vi "Car Wash.vi"() -> ()   [LabVIEW 8.6]
doc: "This VI allows you to simulate a car wash. The wash options controls allow you to determine which cycles will be performed. If none are selected, the High Pressure Wash cycle is the default. Once the start button is clicked, the wash begins. Use the Car Position Simulation control to simulate the position of the vehicle. If the vehicle is in the wrong position for the current cycle, the wash indicators will indicate that and you should change the car position. The Car wash display will give the current status of the wash cycle. The \"Stop Program\" button will stop the car wash immediately."
uses:
  Controls/State Control Enum.ctl
  Controls/Car Wash Indicators.ctl
  Controls/Car Position Control.ctl
  Controls/Wash Options.ctl
panel:
  in  "Stop":bool
  out "Elapsed Time (sec)":dbl format="%#.2g"
  out "Wash Indicators":T1
  in  "Car Position Slider":T2
  out "Wash Entry":bool
  in  "Start":bool
  in  "Wash Options":T3
  # "Entry Console"
  # "Car Wash Display"
  # "The wash options controls allow you to determine which cycles will be performed.  \n\nIf none are selected, the High Pressure Wash cycle is the default.  \n\nOnce the start button is clicked, the wash begins."
  # "The Wash Entry LED indicates whether or not the wash in vacant or in use.\n\nThe Wash Indicator LEDs indicate the current status when the wash is in use.\n\nThe Elapsed Time indicator shows the progress for the current cycle, only if it is a timed cycle."
  # "Car Position Simulation"
  # "The Car Position Slider allows you to simulate the position of a vehicle in the wash.\nThe vehicle must be at the correct station for the each wash cycle to work.  The cycles that are completed at each station are indicated below the station number.\nIf the Vehicle Out of Position LED above is green, adjust your position to the appropraite station."
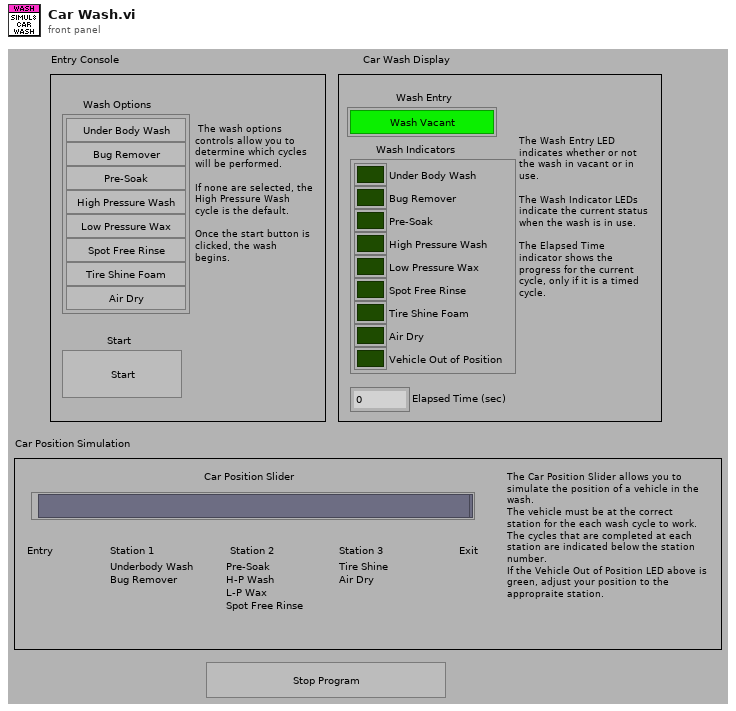
[diagram p1: front panel]
types:
  T1 = typedef "Car Wash Indicators.ctl" = cluster{"Under Body Wash":bool, "Bug Remover":bool, "Pre-Soak":bool, "High Pressure Wash":bool, "Low Pressure Wax":bool, "Spot Free Rinse":bool, "Tire Shine Foam":bool, "Air Dry":bool, "Vehicle Out of Position":bool}
  T2 = typedef "Car Position Control.ctl" = i32
  T3 = typedef "Wash Options.ctl" = cluster{"Under Body Wash":bool, "Bug Remover":bool, "Pre-Soak":bool, "High Pressure Wash":bool, "Low Pressure Wax":bool, "Spot Free Rinse":bool, "Tire Shine Foam":bool, "Air Dry":bool}
  T4 = typedef "State Control Enum.ctl" = enum16{"Initialize", "Wait for Start", "Underbody Wash", "Bug Remover", "Presoak", "HP Wash", "LP Wax", "Spot Free Rinse", "Tire Shine", "Air Dry", "Exit", "Skip", "Stop"}
  T5 = enum8{"Enabled", "Disabled", "Disabled and Grayed Out"}
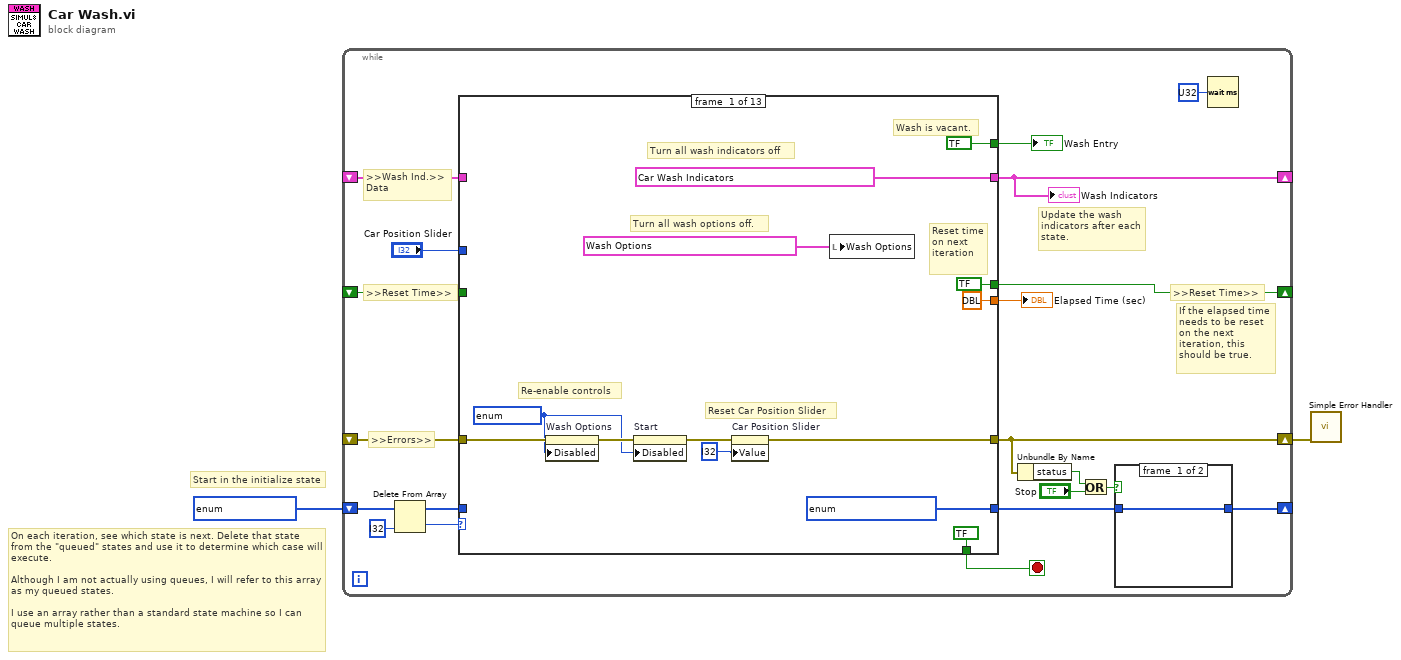
[diagram p0: block diagram]
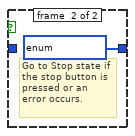
[diagram p2: hidden frame]
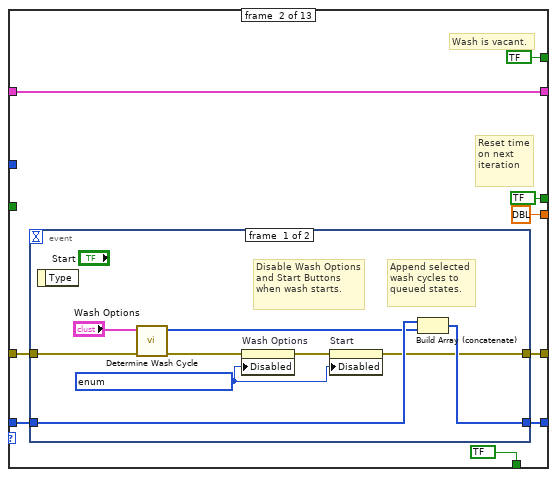
[diagram p3: hidden frame]
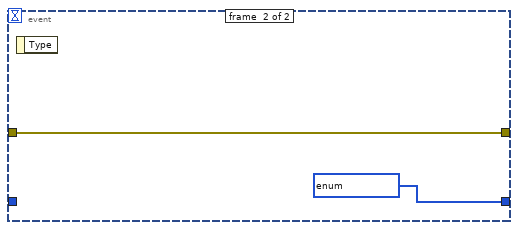
[diagram p4: hidden frame]
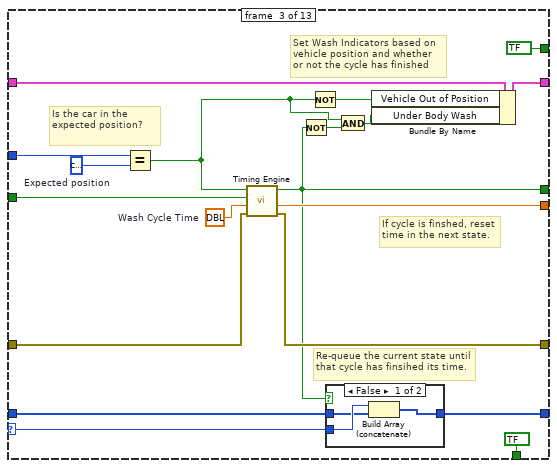
[diagram p5: hidden frame]
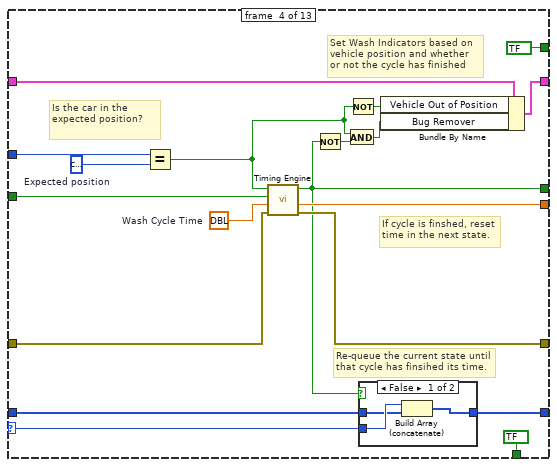
[diagram p7: hidden frame]
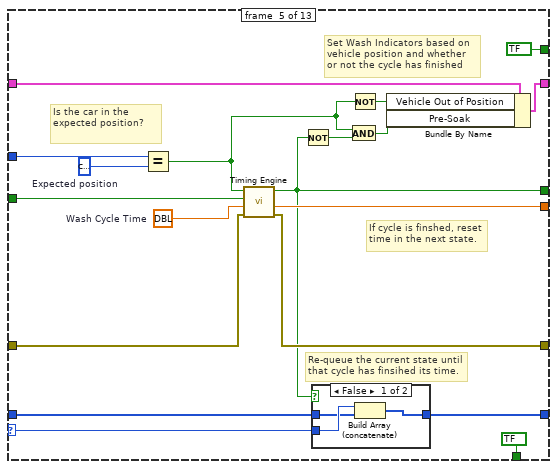
[diagram p9: hidden frame]
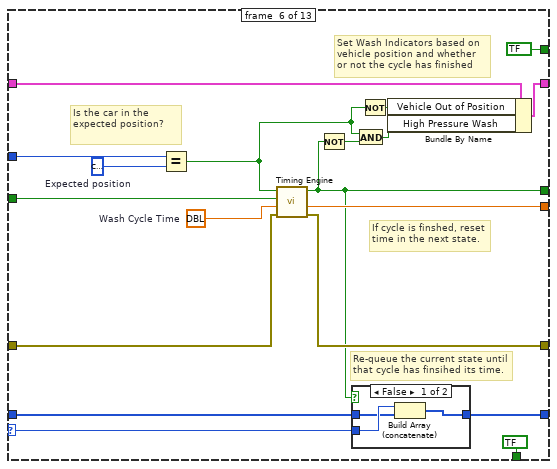
[diagram p11: hidden frame]
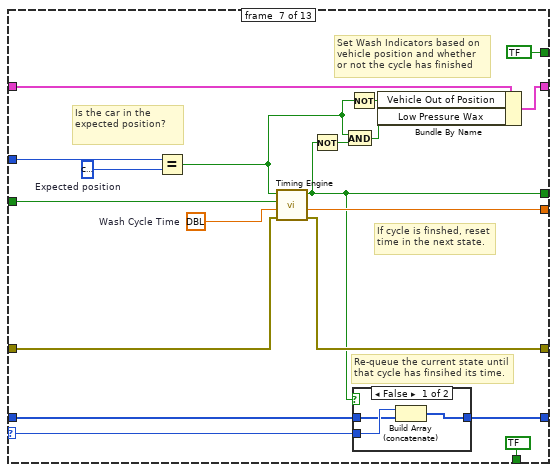
[diagram p13: hidden frame]
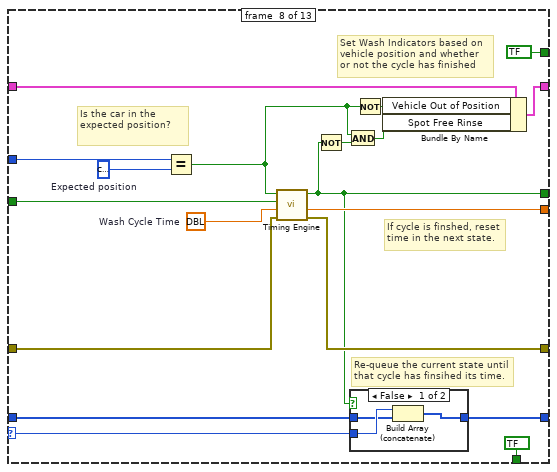
[diagram p15: hidden frame]
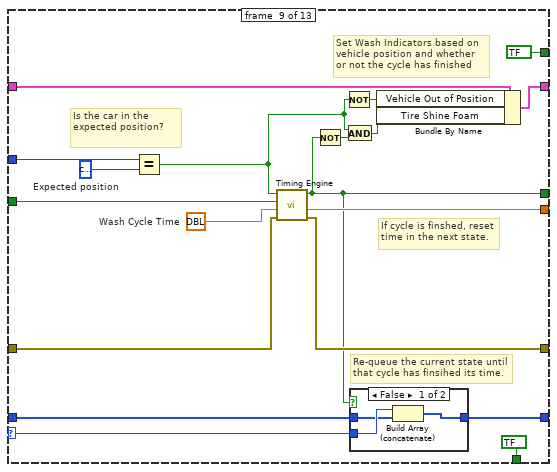
[diagram p17: hidden frame]
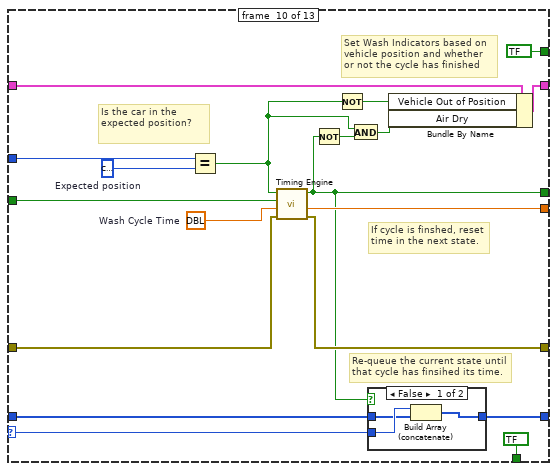
[diagram p19: hidden frame]
diagram:
  w2 = T4[] ? items=["Initialize", "Wait for Start", "Underbody Wash", "Bug Remover", "Presoak", "HP Wash", "LP Wax", "Spot Free Rinse", "Tire Shine", "Air Dry", "Exit", "Skip", "Stop"]
  # "Start in the initialize state"
  # "On each iteration, see which state is next. Delete that state from the \"queued\" states and use it to determine which case will execute. \n\nAlthough I am not actually using queues, I will refer to this array as my queued states.  \n\nI use an array rather than a standard state machine so I can queue multiple states."
  n1 = while {
    shift-right: [w14] -> _
    shift-left: w2 -> [w22]
    shift-right: [w17] -> _
    shift-left: _ -> [w18]
    shift-right: [w6] -> w1
    shift-left: _ -> [w13]
    shift-right: [w12] -> _
    shift-left: _ -> [w11]
    stop <- w8 stop-if-true
    # "Update the wash indicators after each state."
    # "If the elapsed time needs to be reset on the next iteration, this should be true."
    # ">>Reset Time>>"
    # ">>Errors>>"
    # ">>Wash Ind.>>\nData"
    # ">>Reset Time>>"
    n2 = Delete From Array(array=w22, index=i32 ?) -> (deleted portion=w19:T4, array with subset deleted=w20:T4[])  [unwired: 1 in]
    n3 = case shown="\"Air Dry\"" w19 {
      selector: w19 -> [_ _ w65 w90 w114 w143 w159 w188 w204 w232 _ _ _]
      tunnel: w20 -> [_ w44 w64 w91 w115 w142 w158 w187 w203 w231 _ w256 _]
      tunnel: [w29 w45 w66 w89 w113 w141 w157 w180 w205 w230 w243 w256 w270] -> w15
      tunnel: [T1 ? ("Wash Indicators 2") w38 w67 w92 w116 w135 w160 w184 w206 w233 T1 ? ("Wash Indicators 2") w253 w272] -> w17
      tunnel: w18 -> [_ w38 w68 w93 w117 w136 w161 w185 w207 w234 _ w253 w273]
      tunnel: [bool ? ("Wash Entry") bool ? ("Wash Entry") bool ? ("Wash Entry") bool ? ("Wash Entry") bool ? ("Wash Entry") bool ? ("Wash Entry") bool ? ("Wash Entry") bool ? ("Wash Entry") bool ? ("Wash Entry") bool ? ("Wash Entry") bool ? ("Wash Entry") bool ? ("Wash Entry") bool ? ("Wash Entry")] -> w16
      tunnel: w13 -> [w35 w43 w72 w95 w109 w139 w165 w181 w212 w228 w250 w257 w266]
      tunnel: [w25 w42 w73 w94 w110 w140 w164 w189 w211 w229 w249 w258 w266] -> w6
      tunnel: [bool ? ("Time Expired?") bool ? ("Wash Entry") w58 w84 w105 w128 w153 w176 w200 w221 bool ? ("Time Expired?") w260 bool ? ("Time Expired?")] -> w12
      tunnel: w11 -> [_ _ w75 w96 w119 w138 w162 w182 w210 w227 _ w260 _]
      tunnel: [dbl ? ("Elapsed Time") dbl ? ("Elapsed Time") w74 w86 w118 w134 w166 w186 w208 w235 dbl ? ("Elapsed Time") w262 dbl ? ("Elapsed Time")] -> w10
      tunnel: "Car Position Slider" -> [_ _ w70 w97 w120 w137 w163 w183 w209 w226 _ _ w264]
      tunnel: [bool ? ("Wash Entry") bool ? ("Wash Entry") bool ? ("Wash Entry") bool ? ("Wash Entry") bool ? ("Wash Entry") bool ? ("Wash Entry") bool ? ("Wash Entry") bool ? ("Wash Entry") bool ? ("Wash Entry") bool ? ("Wash Entry") bool ? ("Wash Entry") bool ? ("Wash Entry") bool ? ("Wash Entry")] -> w8
      frame #0 {
        w29 = T4[] ? items=["Initialize", "Wait for Start", "Underbody Wash", "Bug Remover", "Presoak", "HP Wash", "LP Wax", "Spot Free Rinse", "Tire Shine", "Air Dry", "Exit", "Skip", "Stop"]
        w26 = T5 ? ("Disabled")
        # "Reset time on next iteration"
        # "Re-enable controls"
        # "Reset Car Position Slider"
        # "Wash is vacant."
        # "Turn all wash indicators off"
        # "Turn all wash options off."
        n4 = property on="Wash Options" class="Clust (strict)"(error in=w35, "Disabled"=w26) -> (error out=w34:errorcluster)  [unwired: 1 in, 1 out]
        n5 = property on="Start" class="Bool"(error in=w34, "Disabled"=w26) -> (error out=w28:errorcluster)  [unwired: 1 in, 1 out]
        n6 = property on="Car Position Slider" class="Slide (strict)"(error in=w28, "Value"=i32 ?) -> (error out=w25:errorcluster)  [unwired: 1 in, 1 out]
        n7 = local write "Wash Options"(T3 ? ("Wash Options")) -> ()
      }
      frame #1 {
        # "Wash is vacant."
        # "Reset time on next iteration"
        n8 = event shown="[1] \"Stop\": Value Change" {
          selector: _ -> [_ _]
          dyn-events: _ -> [_ _]
          timeout: _ -> [_ _]
          tunnel: [w51 w57] -> w45
          tunnel: w44 -> [w53 _]
          tunnel: [w47 w56] -> w42
          tunnel: w43 -> [w48 w56]
          event #0 {
            w49 = T5 ? ("Disabled")
            # "Append selected wash cycles to queued states."
            # "Disable Wash Options and Start Buttons when wash starts."
            n9 = event-data() -> ()  [unwired: 1 in, 1 out]
            n10 = call "Determine Wash Cycle.vi"("error in"=w48, "Wash Options"="Wash Options") -> ("error out"=w54:errorcluster, "Wash Cycles"=w52:T4[])  [unwired: 8 in]
            n11 = property on="Wash Options" class="Clust (strict)"(error in=w54, "Disabled"=w49) -> (error out=w50:errorcluster)  [unwired: 1 in, 1 out]
            n12 = property on="Start" class="Bool"(error in=w50, "Disabled"=w49) -> (error out=w47:errorcluster)  [unwired: 1 in, 1 out]
            n13 = Build Array (concatenate)(w53, w52) -> (w51:T4[])
          }
          event #1 {
            w57 = T4[] ? items=["Initialize", "Wait for Start", "Underbody Wash", "Bug Remover", "Presoak", "HP Wash", "LP Wax", "Spot Free Rinse", "Tire Shine", "Air Dry", "Exit", "Skip", "Stop"]
            n14 = event-data() -> ()  [unwired: 1 in, 1 out]
          }
        }
      }
      frame #2 {
        w69 = T2 ?  # Expected position
        w71 = dbl ?  # Wash Cycle Time
        # "Is the car in the expected position?"
        # "Re-queue the current state until that cycle has finsihed its time."
        # "If cycle is finshed, reset time in the next state."
        # "Set Wash Indicators based on vehicle position and whether or not the cycle has finished"
        n15 = Equal?(x=w70, y=w69) -> (x = y?=w60:bool)
        n16 = call "Timing Engine.vi"("error in"=w72, "Time Limit"=w71, "Reset"=w75, "Advance Time?"=w60) -> ("error out"=w73:errorcluster, "Elapsed Time"=w74:dbl, "Time Expired?"=w58:bool)  [unwired: 5 in]
        n17 = Not(x=w58) -> (.not. x?=w61:bool)
        n18 = Not(x=w60) -> (.not. x?=w63:bool)
        n19 = case shown="False" w58 {
          tunnel: [w79 w80] -> w66
          tunnel: w65 -> [w78 _]
          tunnel: w64 -> [w77 w80]
          frame #0 {
            n20 = Build Array (concatenate)(w78, w77) -> (w79:T4[])
          }
          frame #1 {
          }
        }
        n21 = And(x=w60, y=w61) -> (x .and. y?=w59:bool)
        n22 = Bundle By Name(cluster=w68, "Vehicle Out of Position"=w63, "Under Body Wash"=w59) -> (w67:T1)
      }
      frame #3 {
        w81 = T2 ?  # Expected position
        w98 = dbl ?  # Wash Cycle Time
        # "Is the car in the expected position?"
        # "Re-queue the current state until that cycle has finsihed its time."
        # "If cycle is finshed, reset time in the next state."
        # "Set Wash Indicators based on vehicle position and whether or not the cycle has finished"
        n23 = Equal?(x=w97, y=w81) -> (x = y?=w83:bool)
        n24 = call "Timing Engine.vi"("error in"=w95, "Time Limit"=w98, "Reset"=w96, "Advance Time?"=w83) -> ("error out"=w94:errorcluster, "Elapsed Time"=w86:dbl, "Time Expired?"=w84:bool)  [unwired: 5 in]
        n25 = Not(x=w84) -> (.not. x?=w85:bool)
        n26 = And(x=w83, y=w85) -> (x .and. y?=w82:bool)
        n27 = Not(x=w83) -> (.not. x?=w88:bool)
        n28 = case shown="False" w84 {
          tunnel: [w102 w103] -> w89
          tunnel: w90 -> [w101 _]
          tunnel: w91 -> [w100 w103]
          frame #0 {
            n29 = Build Array (concatenate)(w101, w100) -> (w102:T4[])
          }
          frame #1 {
          }
        }
        n30 = Bundle By Name(cluster=w93, "Vehicle Out of Position"=w88, "Bug Remover"=w82) -> (w92:T1)
      }
      frame #4 {
        w104 = T2 ?  # Expected position
        w121 = dbl ?  # Wash Cycle Time
        # "Is the car in the expected position?"
        # "Re-queue the current state until that cycle has finsihed its time."
        # "If cycle is finshed, reset time in the next state."
        # "Set Wash Indicators based on vehicle position and whether or not the cycle has finished"
        n31 = Equal?(x=w120, y=w104) -> (x = y?=w107:bool)
        n32 = call "Timing Engine.vi"("error in"=w109, "Time Limit"=w121, "Reset"=w119, "Advance Time?"=w107) -> ("error out"=w110:errorcluster, "Elapsed Time"=w118:dbl, "Time Expired?"=w105:bool)  [unwired: 5 in]
        n33 = Not(x=w105) -> (.not. x?=w108:bool)
        n34 = case shown="False" w105 {
          tunnel: [w125 w126] -> w113
          tunnel: w114 -> [w124 _]
          tunnel: w115 -> [w123 w126]
          frame #0 {
            n35 = Build Array (concatenate)(w124, w123) -> (w125:T4[])
          }
          frame #1 {
          }
        }
        n36 = And(x=w107, y=w108) -> (x .and. y?=w106:bool)
        n37 = Not(x=w107) -> (.not. x?=w112:bool)
        n38 = Bundle By Name(cluster=w117, "Vehicle Out of Position"=w112, "Pre-Soak"=w106) -> (w116:T1)
      }
      frame #5 {
        w127 = T2 ?  # Expected position
        w144 = dbl ?  # Wash Cycle Time
        # "Is the car in the expected position?"
        # "Re-queue the current state until that cycle has finsihed its time."
        # "If cycle is finshed, reset time in the next state."
        # "Set Wash Indicators based on vehicle position and whether or not the cycle has finished"
        n39 = Equal?(x=w137, y=w127) -> (x = y?=w129:bool)
        n40 = call "Timing Engine.vi"("error in"=w139, "Time Limit"=w144, "Reset"=w138, "Advance Time?"=w129) -> ("error out"=w140:errorcluster, "Elapsed Time"=w134:dbl, "Time Expired?"=w128:bool)  [unwired: 5 in]
        n41 = Not(x=w128) -> (.not. x?=w131:bool)
        n42 = case shown="False" w128 {
          tunnel: [w148 w149] -> w141
          tunnel: w143 -> [w147 _]
          tunnel: w142 -> [w146 w149]
          frame #0 {
            n43 = Build Array (concatenate)(w147, w146) -> (w148:T4[])
          }
          frame #1 {
          }
        }
        n44 = And(x=w129, y=w131) -> (x .and. y?=w130:bool)
        n45 = Not(x=w129) -> (.not. x?=w133:bool)
        n46 = Bundle By Name(cluster=w136, "Vehicle Out of Position"=w133, "High Pressure Wash"=w130) -> (w135:T1)
      }
      frame #6 {
        w150 = T2 ?  # Expected position
        w167 = dbl ?  # Wash Cycle Time
        # "Is the car in the expected position?"
        # "Re-queue the current state until that cycle has finsihed its time."
        # "If cycle is finshed, reset time in the next state."
        # "Set Wash Indicators based on vehicle position and whether or not the cycle has finished"
        n47 = Equal?(x=w163, y=w150) -> (x = y?=w152:bool)
        n48 = call "Timing Engine.vi"("error in"=w165, "Time Limit"=w167, "Reset"=w162, "Advance Time?"=w152) -> ("error out"=w164:errorcluster, "Elapsed Time"=w166:dbl, "Time Expired?"=w153:bool)  [unwired: 5 in]
        n49 = Not(x=w153) -> (.not. x?=w154:bool)
        n50 = And(x=w152, y=w154) -> (x .and. y?=w151:bool)
        n51 = Not(x=w152) -> (.not. x?=w156:bool)
        n52 = case shown="False" w153 {
          tunnel: [w171 w172] -> w157
          tunnel: w159 -> [w170 _]
          tunnel: w158 -> [w169 w172]
          frame #0 {
            n53 = Build Array (concatenate)(w170, w169) -> (w171:T4[])
          }
          frame #1 {
          }
        }
        n54 = Bundle By Name(cluster=w161, "Vehicle Out of Position"=w156, "Low Pressure Wax"=w151) -> (w160:T1)
      }
      frame #7 {
        w173 = T2 ?  # Expected position
        w190 = dbl ?  # Wash Cycle Time
        # "Is the car in the expected position?"
        # "Re-queue the current state until that cycle has finsihed its time."
        # "If cycle is finshed, reset time in the next state."
        # "Set Wash Indicators based on vehicle position and whether or not the cycle has finished"
        n55 = Equal?(x=w183, y=w173) -> (x = y?=w175:bool)
        n56 = call "Timing Engine.vi"("error in"=w181, "Time Limit"=w190, "Reset"=w182, "Advance Time?"=w175) -> ("error out"=w189:errorcluster, "Elapsed Time"=w186:dbl, "Time Expired?"=w176:bool)  [unwired: 5 in]
        n57 = Not(x=w176) -> (.not. x?=w177:bool)
        n58 = And(x=w175, y=w177) -> (x .and. y?=w174:bool)
        n59 = case shown="False" w176 {
          tunnel: [w194 w195] -> w180
          tunnel: w188 -> [w193 _]
          tunnel: w187 -> [w192 w195]
          frame #0 {
            n60 = Build Array (concatenate)(w193, w192) -> (w194:T4[])
          }
          frame #1 {
          }
        }
        n61 = Not(x=w175) -> (.not. x?=w179:bool)
        n62 = Bundle By Name(cluster=w185, "Vehicle Out of Position"=w179, "Spot Free Rinse"=w174) -> (w184:T1)
      }
      frame #8 {
        w196 = T2 ?  # Expected position
        w213 = dbl ?  # Wash Cycle Time
        # "Is the car in the expected position?"
        # "Re-queue the current state until that cycle has finsihed its time."
        # "If cycle is finshed, reset time in the next state."
        # "Set Wash Indicators based on vehicle position and whether or not the cycle has finished"
        n63 = Equal?(x=w209, y=w196) -> (x = y?=w198:bool)
        n64 = call "Timing Engine.vi"("error in"=w212, "Time Limit"=w213, "Reset"=w210, "Advance Time?"=w198) -> ("error out"=w211:errorcluster, "Elapsed Time"=w208:dbl, "Time Expired?"=w200:bool)  [unwired: 5 in]
        n65 = Not(x=w200) -> (.not. x?=w199:bool)
        n66 = Not(x=w198) -> (.not. x?=w202:bool)
        n67 = And(x=w198, y=w199) -> (x .and. y?=w197:bool)
        n68 = case shown="False" w200 {
          tunnel: [w217 w218] -> w205
          tunnel: w204 -> [w216 _]
          tunnel: w203 -> [w215 w218]
          frame #0 {
            n69 = Build Array (concatenate)(w216, w215) -> (w217:T4[])
          }
          frame #1 {
          }
        }
        n70 = Bundle By Name(cluster=w207, "Vehicle Out of Position"=w202, "Tire Shine Foam"=w197) -> (w206:T1)
      }
      frame #9 {
        w219 = T2 ?  # Expected position
        w236 = dbl ?  # Wash Cycle Time
        # "Is the car in the expected position?"
        # "If cycle is finshed, reset time in the next state."
        # "Re-queue the current state until that cycle has finsihed its time."
        # "Set Wash Indicators based on vehicle position and whether or not the cycle has finished"
        n71 = Equal?(x=w226, y=w219) -> (x = y?=w222:bool)
        n72 = call "Timing Engine.vi"("error in"=w228, "Time Limit"=w236, "Reset"=w227, "Advance Time?"=w222) -> ("error out"=w229:errorcluster, "Elapsed Time"=w235:dbl, "Time Expired?"=w221:bool)  [unwired: 5 in]
        n73 = Not(x=w221) -> (.not. x?=w223:bool)
        n74 = Not(x=w222) -> (.not. x?=w225:bool)
        n75 = And(x=w222, y=w223) -> (x .and. y?=w220:bool)
        n76 = case shown="False" w221 {
          tunnel: [w240 w241] -> w230
          tunnel: w232 -> [w239 _]
          tunnel: w231 -> [w238 w241]
          frame #0 {
            n77 = Build Array (concatenate)(w239, w238) -> (w240:T4[])
          }
          frame #1 {
          }
        }
        n78 = Bundle By Name(cluster=w234, "Vehicle Out of Position"=w225, "Air Dry"=w220) -> (w233:T1)
      }
      frame #10 {
        w243 = T4[] ? items=["Initialize", "Wait for Start", "Underbody Wash", "Bug Remover", "Presoak", "HP Wash", "LP Wax", "Spot Free Rinse", "Tire Shine", "Air Dry", "Exit", "Skip", "Stop"]
        w248 = T5 ? ("Disabled")
        # "Reset time on next iteration"
        # "Reset the car's position to Entry"
        # "Re-enable FP controls"
        n79 = local write "Car Position Slider"(T2 ? ("Car Position Slider")) -> ()
        n80 = property on="Wash Options" class="Clust (strict)"(error in=w250, "Disabled"=w248) -> (error out=w251:errorcluster)  [unwired: 1 in, 1 out]
        n81 = property on="Start" class="Bool"(error in=w251, "Disabled"=w248) -> (error out=w249:errorcluster)  [unwired: 1 in, 1 out]
      }
      frame #11 {
        w254 = dbl ?  # Time Limit
        # "In the skip state, the only action done is to call the timing VI so the timestamp is updated."
        n82 = call "Timing Engine.vi"("error in"=w257, "Time Limit"=w254, "Reset"=w260, "Advance Time?"=bool ?) -> ("error out"=w258:errorcluster, "Elapsed Time"=w262:dbl)  [unwired: 5 in, 1 out]
      }
      frame #12 {
        w263 = T2 ?  # Expected position
        # "Is the car in the expected position?"
        # "Reset time on next iteration"
        # "Stay in the exit position until the car has moved to exit. The go to initialize state."
        n83 = Not Equal?(x=w264, y=w263) -> (x != y?=w271:bool)
        n84 = case shown="True" w271 {
          tunnel: [w274 w275] -> w270
          frame #0 {
            w274 = T4[] ? items=["Initialize", "Wait for Start", "Underbody Wash", "Bug Remover", "Presoak", "HP Wash", "LP Wax", "Spot Free Rinse", "Tire Shine", "Air Dry", "Exit", "Skip", "Stop"]
          }
          frame #1 {
            w275 = T4[] ? items=["Initialize", "Wait for Start", "Underbody Wash", "Bug Remover", "Presoak", "HP Wash", "LP Wax", "Spot Free Rinse", "Tire Shine", "Air Dry", "Exit", "Skip", "Stop"]
          }
        }
        n85 = Bundle By Name(cluster=w273, "Vehicle Out of Position"=w271) -> (w272:T1)
      }
    }
    "Wash Indicators" <- w17
    "Wash Entry" <- w16
    "Elapsed Time (sec)" <- w10
    n86 = Unbundle By Name(w6) -> ("status"=w5:bool)
    n87 = Or(x=w5, y="Stop") -> (x .or. y?=w3:bool)
    n88 = case shown="True" w3 {
      tunnel: w15 -> [w23 _]
      tunnel: [w23 w24] -> w14
      frame #0 {
      }
      frame #1 {
        w24 = T4[] ? items=["Initialize", "Wait for Start", "Underbody Wash", "Bug Remover", "Presoak", "HP Wash", "LP Wax", "Spot Free Rinse", "Tire Shine", "Air Dry", "Exit", "Skip", "Stop"]
        # "Go to Stop state if the stop button is pressed or an error occurs."
      }
    }
    n89 = Wait (ms)(milliseconds to wait=u32 ?) -> ()  [unwired: 1 out]
  }
  n90 = call <vilib>:"Simple Error Handler.vi"("error in (no error)"=w1) -> ()  [unwired: 4 in, 5 out]
